vi "Read ChannelParams.vi"(8 "error in (no error)":errorcluster, 11 "NISTFGenPluginsBase in":refnum<class "NISTFGenPluginsBase.lvclass">) -> (0 "error out":errorcluster, 2 "ChannelParams":T1[](array[typedef]) {"eOutputMode" items=["Function", "Arbitrary", "Sequence"]; "eOperateMode" items=["Continuous", "Burst"]}, 3 "NISTFGenPluginsBase out":refnum<class "NISTFGenPluginsBase.lvclass">)   [LabVIEW 2014, in "FGenPlugins.lvlib" / "NISTFGenPluginsBase.lvclass"]
uses:
  NISTFGenPluginsBase.lvclass
  TypeDef/ChannelParamElement.ctl
  NISTFGenPluginsBase.lvclass/NISTFGenPluginsBase.ctl
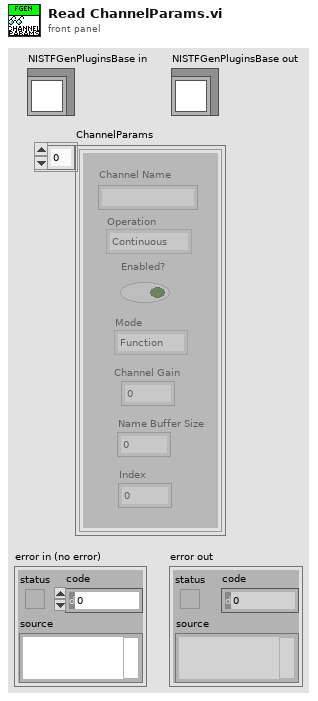
[diagram p1: front panel]
types:
  T1 = typedef "FGenPlugins.lvlib/NISTFGenPluginsBase.lvclass/ChannelParamElement.ctl" = cluster{"sName":string, "eOperateMode":u16, "bEnabled":bool, "eOutputMode":u16, "iIndex":i32, "iNameBufferSize":i32, "fGain":dbl}
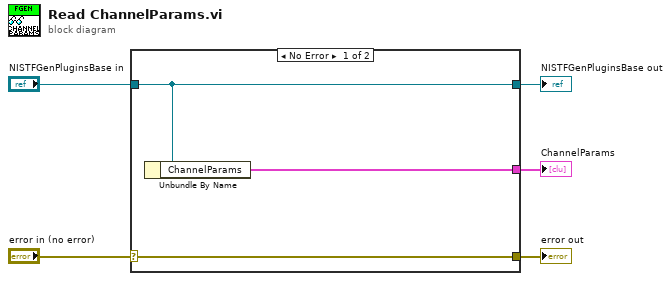
[diagram p0: block diagram]
diagram:
  n1 = case shown="No Error" "error in (no error)" {
    selector: "error in (no error)" -> [w8 w9]
    tunnel: [w8 w9] -> w4
    tunnel: [w7 w10] -> w2
    tunnel: "NISTFGenPluginsBase in" -> [w7 w10]
    tunnel: [w6 _] -> w1
    frame No Error {
      n2 = Unbundle By Name(w7) -> ("ChannelParams"=w6:T1[])
    }
    frame Error {
    }
  }
  "error out" <- w4
  "NISTFGenPluginsBase out" <- w2
  "ChannelParams" <- w1
